vi "RS_RF_send_command.vi"(1 "Value":dbl=3.0, 2 "Parameter":T1(ring), 3 "GPIB address":string="0:19") -> ()   [LabVIEW 2013]
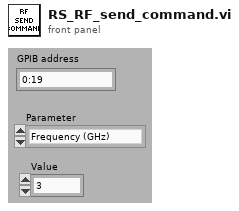
[diagram p1: front panel]
types:
  T1 = enum16{"Frequency (GHz)", "Power (dBm)", "Pulse period (us)", "Pulse width (us)", "Pulse delay (us)", "Pulse modulation?", "Output on?", "Pulse source", "Pulse mode", "Trigger mode", "Ex trigger input slope", "External impedance"}
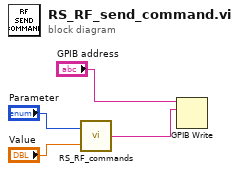
[diagram p0: block diagram]
diagram:
  n1 = call "RS_RF_commands.vi"("Value"="Value", "Parameter"="Parameter") -> ("Command"=w2:string)
  n2 = GPIB Write(0:"GPIB address", 1:w2) -> ()  [unwired: 1 in, 4 out]
